vi "SVFA Zoom Frequency Response (Real-Im).vi"(0 "stimulus signal X [EUx]":waveform(dbl)={"t0"=timestamp(0 s since 1904-01-01), "dt"=1e-05, "Y"=[]}, 1 "response signal Y [EUy]":waveform(dbl)={"t0"=timestamp(0 s since 1904-01-01), "dt"=1e-05, "Y"=[]}, 3 "zoom settings":T7={"frequency range"={"start frequency"=1000.0, "stop frequency"=2000.0}, "window"=1, "number of lines"=400, "% overlap"=0.0} {"% overlap" min=0.0 format="%.2f"; "number of lines" min=2; "window" items=["None ", "Hanning", "Hamming", "Blackman-Harris", "Exact Blackman", "Blackman", "Flat Top", "4 Term B-Harris ", "7 Term B-Harris", "Low Sidelobe"]; "frequency range"."stop frequency" min=0.0 format="%.2f"; "frequency range"."start frequency" min=0.0 format="%.2f"}, 5 "error in (no error)":errorcluster, 6 "FRF mode":enum16{"H1", "H2", "H3"}(ring), 7 "averaging parameters":T8={"averaging mode"=enum."No averaging", "weighting mode"=enum."Exponential", "number of averages"=10, "linear mode"=enum."One shot"} {"number of averages" min=1 step=1}, 9 "restart averaging (F)":bool) -> (10 "new spectrum available":bool, 11 "averaging done":bool, 12 "coherence":cluster{"f0":dbl, "df":dbl, "coherence":dbl[]}={"f0"=1001.2500000000001, "df"=2.4999999999999996, "coherence"=[]} {"coherence" format="%.2p"; "df" format="%.2p"; "f0" format="%.2p"}, 13 "averages completed":dbl, 14 "real part [EUy/EUx rms]":cluster{"f0":dbl, "df":dbl, "real part":dbl[]}={"f0"=1001.2500000000001, "df"=2.4999999999999996, "real part"=[]} {"real part" format="%.2p"; "df" format="%.2p"; "f0" format="%.2p"}, 16 "imaginary part [EUy/EUx rms]":T9={"f0"=1001.2500000000001, "df"=2.4999999999999996, "imaginary part"=[]} {"imaginary part" format="%.2p"; "df" format="%.2p"; "f0" format="%.2p"}, 17 "unit label":string=" rms", 18 "spectrum info":T1={"channel name"="", "description"="", "x-axis units"=1, "spectral info"={"spectrum type"=enum."Power [Magnitude^2]", "linear/dB"=enum."linear", "window"=0, "window size"=0, "FFT size"=0}, "engineering units"=0, "custom label"="", "dB reference [EU]"=0.0, "peak units"=enum."rms", "weighting filter"=0, "spectral density?"=FALSE, "unit label"="", "spectrum skewed?"=FALSE, "complimentary spectrum units"=enum."none"} {"x-axis units" items=["Time (s)"=0, "Frequency-CB (Hz)"=1, "Frequency-CPB (Hz)"=1248, "Frequency-Arbitrary (Hz)"=2357, "Quefrency (s)"=2, "Revolutions (rev)"=3, "Order"=4, "Speed (RPM)"=11, "Speed (rad/s)"=21, "Index"=65535]; "weighting filter" items=["Linear", "A-weighting", "B-weighting", "C-weighting", "ITU-R 468-4", "Dolby", "CCITT", "C-message", "Wb", "Wc", "Wd", "We", "Wf", "Wh", "Wj", "Wk", "Wm", "AES17 20 kHz lowpass", "AES17 40 kHz lowpass", "AES17 20 kHz highpass", "AES17 40 kHz highpass"]; "dB reference [EU]" format="%.2f"; "engineering units" items=["custom..."=0, "V"=1, "A"=21, "C"=30, "pC"=31, "s"=32, "-"=29, "Pa"=2, "N"=20, "g"=3, "m/s^2"=4, "m/s"=5, "m"=6, "mm/s"=12, "mm"=13, "micron/s"=14, "micron"=15, "in/s^2"=7, "in/s"=8, "in"=9, "mil/s"=10, "mil"=11, "rad/s^2"=16, "rad/s"=17, "rad"=18, "deg/s^2"=26, "deg/s"=27, "deg"=28, "RPM"=22, "cycle/s^2"=23, "Hz"=24, "cycle"=25, "strain"=19]; "spectral info"."window" items=["None "=0, "Hanning"=1, "Hamming"=2, "Blackman-Harris"=3, "Exact Blackman"=4, "Blackman"=5, "Flat Top"=6, "4 Term B-Harris "=7, "7 Term B-Harris"=8, "Low Sidelobe"=9, "Force - Exponential"=10, "Gaussian"=62]}, 19 "error out":errorcluster)   [LabVIEW 2017]
doc: "Computes the zoom frequency response and the coherence of <B>stimulus signal X [EUx]</B>, <B>response signal Y [EUy]</B>, and <B>zoom settings</B>. Results are returned in coherence, real part, and imaginary part. Data accumulates each time this VI is called. However, it returns a new spectrum only when sufficient data accumulates. Indicators and subsequent processing should only be called when <B>new spectrum available</B> is TRUE.\n\nZoom frequency response is typically an averaged measurement."
uses:
  <vilib>/addons/_NISVFA/_Shared subVIs/Controls/svc_Spectrum Info.ctl
  <vilib>/addons/_NISVFA/_Shared subVIs/Controls/svc_X-Axis Units.ctl
  <vilib>/addons/_NISVFA/_Shared subVIs/Controls/svc_Spectrum Type.ctl
  <vilib>/addons/_NISVFA/_Shared subVIs/Controls/svc_Engineering Units Text Ring.ctl
  <vilib>/addons/_NISVFA/_Shared subVIs/Controls/svc_Weighting Filter Text Ring.ctl
  <vilib>/addons/_NISVFA/_Shared subVIs/Controls/svc_Complimentary Spectrum Units.ctl
  <vilib>/addons/_NISVFA/_Shared subVIs/Spectrum Averaging/svfa_Reset Averaging State Info.vi
  <vilib>/addons/_NISVFA/_Shared subVIs/Spectrum Averaging/svfa_Average Array with Avg Checks (complex) No State.vi
  <vilib>/addons/_NISVFA/_Shared subVIs/Spectrum Averaging/svfa_Average Spectrum (complex) No State.vi
  <vilib>/addons/_NISVFA/_Shared subVIs/Spectrum Averaging/svfa_Average Array (complex) No State.vi
  <vilib>/addons/_NISVFA/_Shared subVIs/Spectrum Averaging/svfa_No Average Array (complex).vi
  <vilib>/addons/_NISVFA/_Shared subVIs/Spectrum Averaging/svfa_Average Array (complex).vi
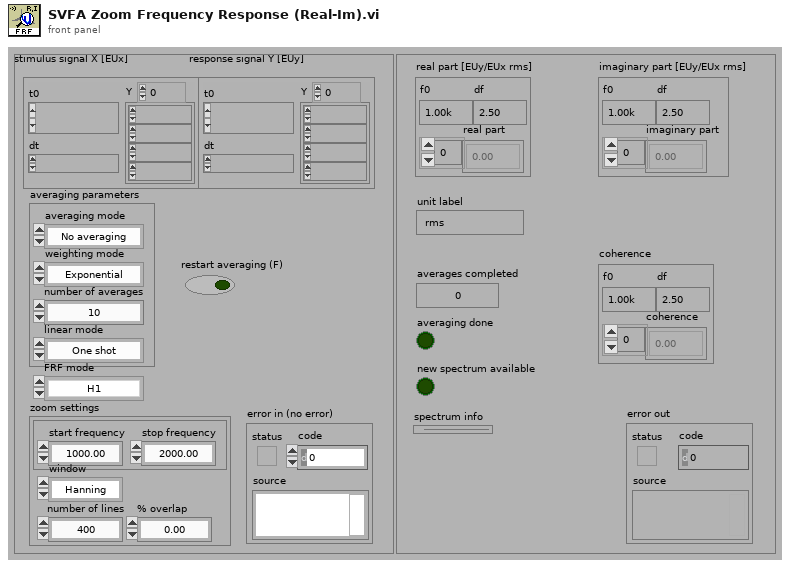
[diagram p1: front panel]
types:
  T1 = typedef "svc_Spectrum Info.ctl" = cluster{"channel name":string, "description":string, "x-axis units":T2, "spectral info":cluster{"spectrum type":T3, "linear/dB":enum16{"linear", "dB"}, "window":u16, "window size":i32, "FFT size":i32}, "engineering units":T4, "custom label":string, "dB reference [EU]":dbl, "peak units":enum16{"rms", "peak", "peak-peak"}, "weighting filter":T5, "spectral density?":bool, "unit label":string, "spectrum skewed?":bool, "complimentary spectrum units":T6}
  T2 = typedef "svc_X-Axis Units.ctl" = u16
  T3 = typedef "svc_Spectrum Type.ctl" = enum16{"FFT Spectrum [complex]", "Amplitude [Magnitude]", "Power [Magnitude^2]", "Cross Spectrum [complex]", "Frequency Response [Complex]"}
  T4 = typedef "svc_Engineering Units Text Ring.ctl" = u16
  T5 = typedef "svc_Weighting Filter Text Ring.ctl" = u16
  T6 = typedef "svc_Complimentary Spectrum Units.ctl" = enum16{"none", "radians", "degrees", "cycles", "imaginary"}
  T7 = cluster{"frequency range":cluster{"start frequency":dbl, "stop frequency":dbl}, "window":u16, "number of lines":i32, "% overlap":dbl}
  T8 = cluster{"averaging mode":enum16{"No averaging", "Vector averaging", "RMS averaging", "Peak hold"}, "weighting mode":enum16{"Linear", "Exponential"}, "number of averages":u32, "linear mode":enum16{"One shot", "Auto restart"}}
  T9 = cluster{"f0":dbl, "df":dbl, "imaginary part":dbl[]}
  T10 = enum16{"Cross spectrum", "Frequency response", "Coherent output power"}
  T11 = enum16{"Restart processing", "Continue processing", "Skip processing"}
  T12 = enum16{"No averaging", "Vector averaging", "RMS averaging", "Peak hold"}
  T13 = cluster{"zoom settings":cluster{"center frequency":dbl, "zoom":i32, "trim":dbl}, "FFT settings":cluster{"window":enum16{"None ", "Hanning", "Hamming", "Blackman-Harris", "Exact Blackman", "Blackman", "Flat Top", "4 Term B-Harris ", "7 Term B-Harris", "Low Sidelobe"}, "window size":i32, "FFT size":i32, "%overlap":dbl}}
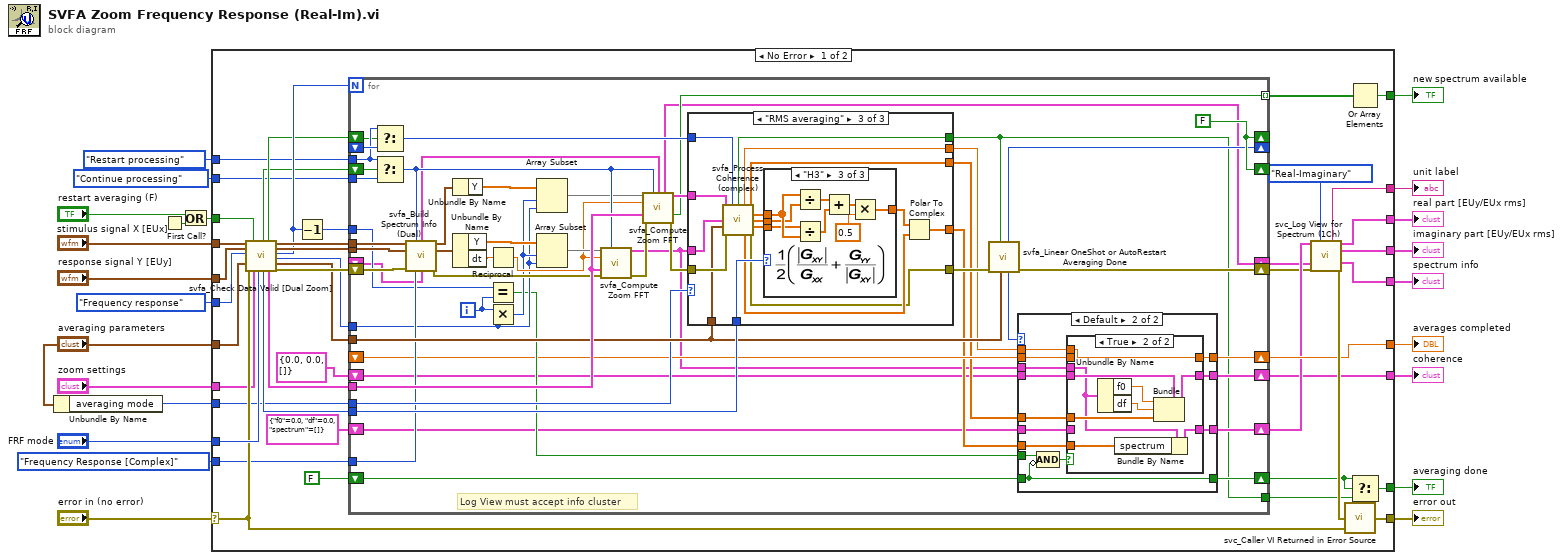
[diagram p0: block diagram]
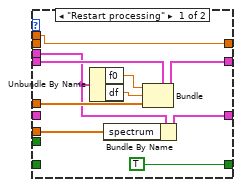
[diagram p2: hidden frame]
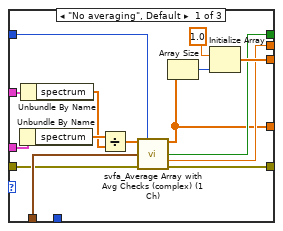
[diagram p4: hidden frame]
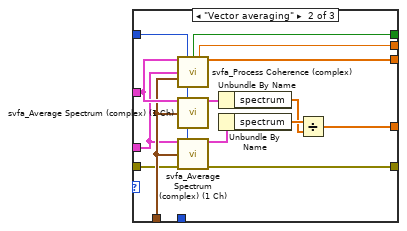
[diagram p5: hidden frame]
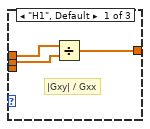
[diagram p6: hidden frame]
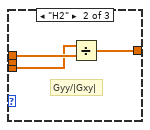
[diagram p7: hidden frame]
diagram:
  # "Log View must accept info cluster"
  n1 = Unbundle By Name("averaging parameters") -> ("averaging mode"=w10:T12)
  n2 = First Call?() -> (First Call?: T/F=w23:bool)
  n3 = Or(x="restart averaging (F)", y=w23) -> (x .or. y?=w19:bool)
  n4 = case shown="No Error" "error in (no error)" {
    selector: "error in (no error)" -> [w55 w214]
    tunnel: "stimulus signal X [EUx]" -> [w66 _]
    tunnel: "response signal Y [EUy]" -> [w65 _]
    tunnel: [w62 _] -> w3
    tunnel: [w61 _] -> w2
    tunnel: [w47 _] -> w6
    tunnel: [w56 w214] -> w8
    tunnel: [w25 _] -> w1
    tunnel: w19 -> [w63 _]
    tunnel: "zoom settings" -> [w53 _]
    tunnel: [w27 _] -> w9
    tunnel: [w50 _] -> w5
    tunnel: [w60 _] -> w7
    tunnel: "FRF mode" -> [w59 _]
    tunnel: [w58 _] -> w4
    tunnel: "averaging parameters" -> [w64 _]
    tunnel: T10."Frequency response" ("measurement") -> [w52 _]
    tunnel: svc_Spectrum_Type."Frequency Response [Complex]" ("spectrum type") -> [w37 _]
    tunnel: w10 -> [w36 _]
    tunnel: T11."Restart processing" ("processing control") -> [w33 _]
    tunnel: T11."Continue processing" ("processing control") -> [w32 _]
    frame No Error {
      n5 = call <vilib>:"svfa_Check Data Valid [Dual Zoom].vi"("stimulus [X]"=w66, "response [Y]"=w65, "measurement"=w52, "averaging parameters"=w64, "error in (no error)"=w55, "restart averaging (F)"=w63, "zoom settings"=w53, "FRF mode"=w59) -> ("reset processing"=w34:bool, "dup FRF mode"=w41:enum16{"H1", "H2", "H3"}, "restart averaging"=w35:bool, "zoom FFT settings"=w38:T13, "dup stimulus [X]"=w45:waveform(dbl), "dup response [Y]"=w44:waveform(dbl), "iterations"=w40:i32, "maximum block size"=w31:i32, "dup averaging parameters"=w42:T8, "error out"=w43:errorcluster)  [unwired: 2 in]
      n6 = Decrement(x=w40) -> (x-1=w39:i32)
      n7 = for {
        N: w40 -> [_]
        shift-left: cluster{"f0":dbl, "df":dbl, "Coherence":dbl[]} {"f0"=0.0, "df"=0.0, "Coherence"=[]} -> [w73]
        shift-right: [w77] -> w47
        shift-left: cluster{"f0":dbl, "df":dbl, "spectrum":cdb[]} {"f0"=0.0, "df"=0.0, "spectrum"=[]} ("FFT spectrum") -> [w72]
        shift-right: [w74] -> w49
        tunnel: w42 -> [w112]
        tunnel: [w67] -> w24
        tunnel: [w71] -> w51 mode=indexing
        tunnel: w41 -> [w114]
        tunnel: w44 -> [w108]
        tunnel: w45 -> [w109]
        shift-right: [w69] -> w48
        shift-left: _ -> [w68]
        shift-right: [w85] -> _
        shift-left: _ -> [w100]
        tunnel: w39 -> [w93]
        tunnel: w38 -> [w118]
        tunnel: w37 -> [w103]
        tunnel: w36 -> [w110]
        shift-right: [w119] -> w46
        shift-left: w43 -> [w104]
        shift-right: [w81] -> w50
        shift-left: _ -> [w80]
        shift-right: [w95] -> _
        shift-left: w35 -> [w98]
        shift-right: [w95] -> _
        shift-left: w34 -> [w102]
        tunnel: w33 -> [w99]
        tunnel: w32 -> [w101]
        tunnel: w31 -> [w86]
        shift-right: [w83] -> w26
        shift-left: FALSE ("restart averaging") -> [w82]
        i -> [w94]
        w95 = FALSE ("reset processing")
        n8 = Select(t=w99, s=w98, f=w100) -> (s? t:f=w96:T11)
        n9 = Select(t=w99, s=w102, f=w101) -> (s? t:f=w97:T11)
        n10 = call <vilib>:"svfa_Build Spectrum Info (Dual).vi"("scaled signal  X [EU]"=w109, "processing control"=w97, "scaled signal  Y [EU]"=w108, "error in (no error)"=w104, "spectrum type"=w103, "spectrum info in"=w68) -> ("spectrum info out"=w70:T1, "dup scaled signal  X [EU]"=w107:waveform(dbl), "dup scaled signal  Y [EU]"=w106:waveform(dbl), "error out"=w105:errorcluster)  [unwired: 5 in, 1 out]
        n11 = Unbundle By Name ("Get Waveform Components")(w107) -> ("Y"=w92:dbl[])
        n12 = Unbundle By Name ("Get Waveform Components")(w106) -> ("Y"=w90:dbl[], "dt"=w117:dbl)
        n13 = Reciprocal(x=w117) -> (1/x=w88:dbl)
        n14 = Equal?(x=w93, y=w94) -> (x = y?=w84:bool)
        n15 = Multiply(x=w94, y=w86) -> (x*y=w87:i32)
        n16 = Array Subset(array=w92, index=w87, length=w86) -> (w91:dbl[])
        n17 = Array Subset(array=w90, index=w87, length=w86) -> (w89:dbl[])
        n18 = call <vilib>:"svfa_Compute Zoom FFT.vi"("x"=w89, "processing control"=w97, "fs"=w88, "zoom FFT settings"=w118, "error in (no error)"=w105) -> ("FFT spectrum"=w75:cluster{"f0":dbl, "df":dbl, "spectrum":cdb[]}, "error out"=w116:errorcluster)  [unwired: 6 in, 3 out]
        n19 = call <vilib>:"svfa_Compute Zoom FFT.vi"("x"=w91, "processing control"=w97, "spectrum info"=w70, "fs"=w88, "zoom FFT settings"=w118, "error in (no error)"=w116) -> ("spectrum info out"=w69:T1, "FFT spectrum"=w113:cluster{"f0":dbl, "df":dbl, "spectrum":cdb[]}, "spectrum ready"=w71:bool, "error out"=w115:errorcluster)  [unwired: 5 in, 1 out]
        n20 = case shown="\"RMS averaging\"" w110 {
          tunnel: [w157 w173 w186] -> w111
          tunnel: w112 -> [w161 w177 w197]
          tunnel: [w160 w180 w195] -> w67
          tunnel: w113 -> [w168 w182 w187]
          tunnel: w75 -> [w164 w175 w188]
          tunnel: w115 -> [w158 w174 w198]
          tunnel: w114 -> [_ _ w196]
          tunnel: [w159 w179 w194] -> w79
          tunnel: w96 -> [w156 w176 w193]
          tunnel: [w163 w171 w185] -> w78
          tunnel: [w155 w170 w184] -> w76
          frame "No averaging", Default {
            n21 = Unbundle By Name(w164) -> ("spectrum"=w169:cdb[])
            n22 = Unbundle By Name(w168) -> ("spectrum"=w166:cdb[])
            n23 = Divide(x=w169, y=w166) -> (x/y=w162:cdb[])
            n24 = call <vilib>:"svfa_Average Array with Avg Checks (complex) (1 Ch).vi"("spectrum"=w162, "processing control"=w156, "averaging parameters"=w161, "error in (no error)"=w158) -> ("average spectrum"=w155:cdb[], "averaging done"=w160:bool, "averages completed"=w159:dbl, "error out"=w157:errorcluster)  [unwired: 7 in, 1 out]
            n25 = Array Size(array=w155) -> (size(s)=w165:i32)
            n26 = Initialize Array(1.0 ("overwrite value"), w165) -> (w163:dbl[])
          }
          frame "Vector averaging" {
            n27 = call <vilib>:"svfa_Process Coherence (complex).vi"("X FFT spectrum [Vrms]"=w182, "processing control"=w176, "Y FFT spectrum [Vrms]"=w175, "averaging parameters"=w177) -> ("averaging done"=w180:bool, "averages completed"=w179:dbl, "Coherence"=w171:dbl[])  [unwired: 4 in, 5 out]
            n28 = call <vilib>:"svfa_Average Spectrum (complex) (1 Ch).vi"("spectrum"=w182, "processing control"=w176, "averaging parameters"=w177) -> ("spectrum"=w181:cluster{"f0":dbl, "df":dbl, "spectrum":cdb[]})  [unwired: 8 in, 4 out]
            n29 = call <vilib>:"svfa_Average Spectrum (complex) (1 Ch).vi"("spectrum"=w175, "processing control"=w176, "averaging parameters"=w177, "error in (no error)"=w174) -> ("spectrum"=w172:cluster{"f0":dbl, "df":dbl, "spectrum":cdb[]}, "error out"=w173:errorcluster)  [unwired: 7 in, 3 out]
            n30 = Unbundle By Name(w181) -> ("spectrum"=w178:cdb[])
            n31 = Unbundle By Name(w172) -> ("spectrum"=w183:cdb[])
            n32 = Divide(x=w183, y=w178) -> (x/y=w170:cdb[])
          }
          frame "RMS averaging" {
            n33 = call <vilib>:"svfa_Process Coherence (complex).vi"("X FFT spectrum [Vrms]"=w187, "processing control"=w193, "Y FFT spectrum [Vrms]"=w188, "averaging parameters"=w197, "error in (no error)"=w198) -> ("averaging done"=w195:bool, "averages completed"=w194:dbl, "Coherence"=w185:dbl[], "MAG <Gxy>"=w191:dbl[], "<Gxx>"=w190:dbl[], "<Gyy>"=w189:dbl[], "PHASE <Gxy>"=w192:dbl[], "error out"=w186:errorcluster)  [unwired: 3 in]
            n34 = case shown="\"H3\"" w196 {
              tunnel: w189 -> [_ w203 w206]
              tunnel: [w202 w205 w213] -> w199
              tunnel: w190 -> [w200 _ w207]
              tunnel: w191 -> [w201 w204 w208]
              frame "H1", Default {
                # "|Gxy| / Gxx"
                n35 = Divide(x=w201, y=w200) -> (x/y=w202:dbl[])
              }
              frame "H2" {
                # "Gyy/|Gxy|"
                n36 = Divide(x=w203, y=w204) -> (x/y=w205:dbl[])
              }
              frame "H3" {
                n37 = Divide(x=w208, y=w207) -> (x/y=w209:dbl[])
                n38 = Divide(x=w206, y=w208) -> (x/y=w210:dbl[])
                n39 = Add(x=w209, y=w210) -> (x+y=w211:dbl[])
                n40 = Multiply(x=w211, y=0.5) -> (x*y=w213:dbl[])
              }
            }
            n41 = Polar To Complex(1:w192, 2:w199) -> (0:w184:cdb[])
          }
        }
        n42 = call <vilib>:"svfa_Linear OneShot or AutoRestart Averaging Done.vi"("averaging parameters"=w112, "averaging done"=w67, "error in (no error)"=w111) -> ("error out"=w119:errorcluster, "processing control"=w85:T11)  [unwired: 7 in]
        n43 = case shown="Default" w85 {
          tunnel: [TRUE ("restart averaging") w140] -> w83
          tunnel: w82 -> [_ w140]
          tunnel: w84 -> [_ w142]
          tunnel: [w128 w139] -> w81
          tunnel: w80 -> [_ w138]
          tunnel: w79 -> [w128 w137]
          tunnel: w78 -> [w127 w136]
          tunnel: w75 -> [w120 w130]
          tunnel: [w123 w135] -> w77
          tunnel: w73 -> [w124 w132]
          tunnel: w76 -> [w122 w133]
          tunnel: [w121 w134] -> w74
          tunnel: w72 -> [_ w131]
          frame "Restart processing" {
            n44 = Unbundle By Name(w120) -> ("f0"=w125:dbl, "df"=w126:dbl)
            n45 = Bundle By Name(cluster=w120, "spectrum"=w122) -> (w121:cluster{"f0":dbl, "df":dbl, "spectrum":cdb[]})
            n46 = Bundle(cluster=w124, "f0"=w125, "df"=w126, "Coherence"=w127) -> (w123:cluster{"f0":dbl, "df":dbl, "Coherence":dbl[]})
          }
          frame Default {
            n47 = Compound Arithmetic op=AND(w142, invert w140) -> (w141:bool)
            n48 = case shown="True" w141 {
              tunnel: [w145 w154] -> w139
              tunnel: w138 -> [w145 _]
              tunnel: w137 -> [_ w154]
              tunnel: w130 -> [_ w146]
              tunnel: w136 -> [_ w151]
              tunnel: [w144 w147] -> w135
              tunnel: [w143 w150] -> w134
              tunnel: w133 -> [_ w149]
              tunnel: w132 -> [w144 w148]
              tunnel: w131 -> [w143 _]
              frame False {
              }
              frame True {
                n49 = Unbundle By Name(w146) -> ("f0"=w152:dbl, "df"=w153:dbl)
                n50 = Bundle By Name(cluster=w146, "spectrum"=w149) -> (w150:cluster{"f0":dbl, "df":dbl, "spectrum":cdb[]})
                n51 = Bundle(cluster=w148, "f0"=w152, "df"=w153, "Coherence"=w151) -> (w147:cluster{"f0":dbl, "df":dbl, "Coherence":dbl[]})
              }
            }
          }
        }
      }
      n52 = call <vilib>:"svc_Log View for Spectrum (1Ch).vi"("complex spectrum"=w49, "View"=enum16{"Mag-Phase", "Real-Imaginary"}."Real-Imaginary", "spectrum info in"=w48, "error in (no error)"=w46) -> ("unit label [mag or real]"=w58:string, "magnitude or real"=w62:cluster{"f0":dbl, "df":dbl, dbl[]}, "phase or imag"=w61:cluster{"f0":dbl, "df":dbl, dbl[]}, "spectrum info out"=w60:T1, "error out"=w57:errorcluster)  [unwired: 6 in, 1 out]
      n53 = call <vilib>:"svc_Caller VI Returned in Error Source.vi"("warning input to caller"=w55, "error in (no error)"=w57) -> ("error out"=w56:errorcluster)  [unwired: 3 in]
      n54 = Or Array Elements(Boolean array=w51) -> (logical OR=w27:bool)
      n55 = Select(t=w26, s=w26, f=w24) -> (s? t:f=w25:bool)
    }
    frame Error {
    }
  }
  "error out" <- w8
  "real part [EUy/EUx rms]" <- w3
  "imaginary part [EUy/EUx rms]" <- w2
  "averaging done" <- w1
  "averages completed" <- w5
  "coherence" <- w6
  "new spectrum available" <- w9
  "spectrum info" <- w7
  "unit label" <- w4
